vi "Retrieve All Tables.vi"(8 "error in (no error)":errorcluster, 11 "xwpfReader in":refnum<class "xwpfReader.lvclass">) -> (0 "error out":errorcluster, 2 "Tables":string[][][](array[string]), 3 "xwpfReader out":refnum<class "xwpfReader.lvclass">)   [LabVIEW 2017, in "xwpfReader.lvclass"]
doc: "Retrieves all the Table contents from the document. \n\nThis VI iterates through each table (rows and columns) to get their contents."
uses:
  xwpfReader.lvclass
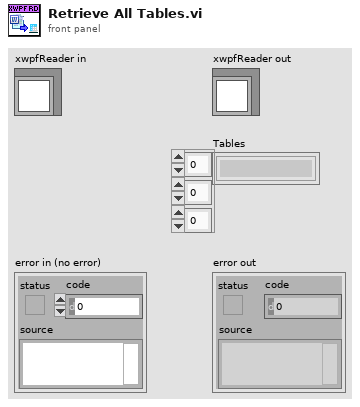
[diagram p1: front panel]
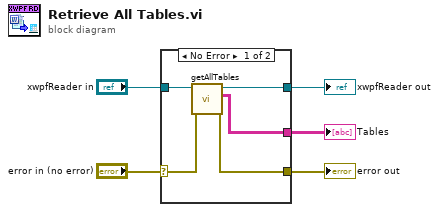
[diagram p0: block diagram]
diagram:
  n1 = case shown="No Error" "error in (no error)" {
    selector: "error in (no error)" -> [w8 w12]
    tunnel: [w7 w12] -> w4
    tunnel: [w9 w11] -> w2
    tunnel: "xwpfReader in" -> [w10 w11]
    tunnel: [w6 _] -> w1
    frame No Error {
      n2 = call "getAllTables.vi"("error in (no error)"=w8, "xwpfReader in"=w10) -> ("error out"=w7:errorcluster, "Tables"=w6:string[][][], "xwpfReader out"=w9:refnum<class "xwpfReader.lvclass">)  [unwired: 7 in]
    }
    frame Error {
    }
  }
  "error out" <- w4
  "xwpfReader out" <- w2
  "Tables" <- w1
